vi "Rename Child Nodes to Default Class Name.vi"(8 "error in (no error)":errorcluster, 11 "DataNode*":refnum<data-value>) -> (0 "error out":errorcluster, 3 "DataNode* Out":refnum<data-value>)   [LabVIEW 2013, in "FPGADMAChannelData.lvclass"]
uses:
  FPGADMAChannelData.lvclass
  xCE/xceDataNode/xceDataNode.lvclass
  xCE/xceNode/xceNode.lvclass
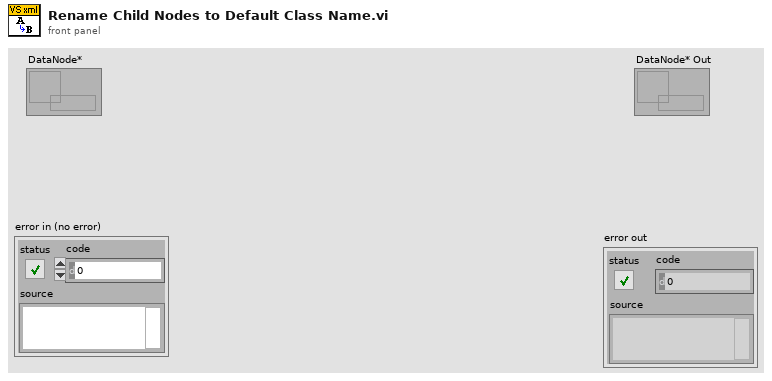
[diagram p1: front panel]
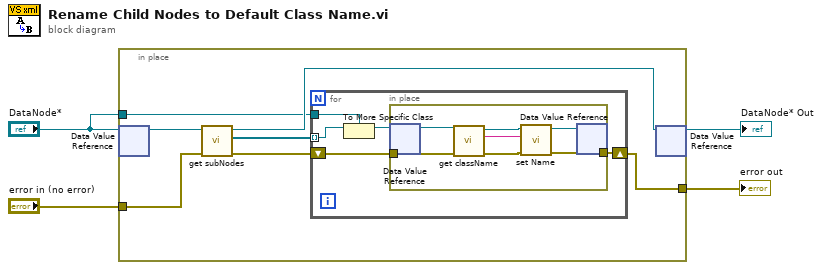
[diagram p0: block diagram]
diagram:
  n1 = in-place {
    in-place-border: "error in (no error)" -> [w5]
    in-place-border: "DataNode*" -> [w9]
    in-place-border: [w6] -> w1
    n2 = in-place-dvr #1("DataNode*") -> (w8:refnum<class "xceDataNode.lvclass">)  [unwired: 1 out]
    n3 = call "get subNodes.vi"("error in (no error)"=w5, "xceNode in"=w8) -> ("error out"=w7:errorcluster, "subNodes[]*"=w11:refnum<data-value>[], "xceNode out"=w10:refnum<class "xceDataNode.lvclass">)  [unwired: 7 in]
    n4 = for {
      tunnel: w11 -> [w15] mode=indexing
      tunnel: w9 -> [w16]
      shift-right: [w12] -> w6
      shift-left: w7 -> [w13]
      n5 = To More Specific Class(target class=w16, reference=w15) -> (specific class reference=w14:refnum<data-value>)  [unwired: 1 in, 1 out]
      n6 = in-place {
        in-place-border: w13 -> [w20]
        in-place-border: [w18] -> w12
        n7 = in-place-dvr #2(w14) -> (w23:refnum<class "xceDataNode.lvclass">)  [unwired: 1 out]
        n8 = call "get className.vi"("error in (no error)"=w20, "xceNode in"=w23) -> ("error out"=w19:errorcluster, "Class name"=w21:string, "xceNode out"=w22:refnum<class "xceDataNode.lvclass">)  [unwired: 7 in]
        n9 = call "set Name.vi"("error in (no error)"=w19, "Name"=w21, "xceDataNode in"=w22) -> ("error out"=w18:errorcluster, "xceDataNode out"=w17:refnum<class "xceDataNode.lvclass">)  [unwired: 7 in]
        n10 = in-place-dvr #2(w17) -> ()  [unwired: 2 out]
      }
    }
    n11 = in-place-dvr #1(w10) -> (→"DataNode* Out":refnum<data-value>)  [unwired: 1 out]
  }
  "error out" <- w1
